vi "shared variable test.vi"() -> ()   [LabVIEW 2019]
panel:
  in  "stop":bool
  out "error out":errorcluster
  out "Email155":string[](array[string])
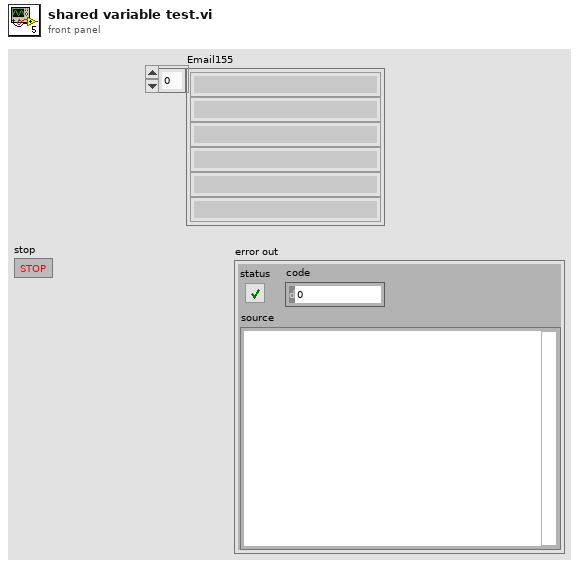
[diagram p1: front panel]
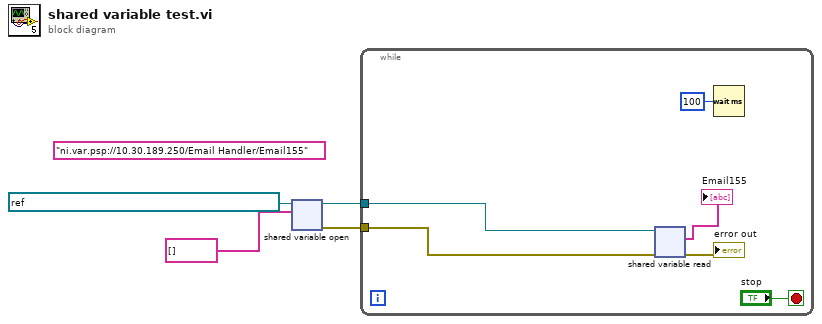
[diagram p0: block diagram]
diagram:
  (unwired) "ni.var.psp://10.30.189.250/Email Handler/Email155" ("format string")
  n1 = shared-variable-open(refnum<k21> "ni.var.psp://localhost/Email Handler/Email155" ("shared variable refnum in"), string[] [] ("data type")) -> (w3:refnum<k21>, w1:errorcluster)  [unwired: 2 in]
  n2 = while {
    tunnel: w3 -> [w6]
    tunnel: w1 -> [w5]
    stop <- "stop" stop-if-true
    n3 = shared-variable-read(w6, w5) -> (→"error out":errorcluster, →"Email155":string[])  [unwired: 2 out]
    n4 = Wait (ms)(milliseconds to wait=u32 100) -> ()  [unwired: 1 out]
  }
